vi "ImgCtrl.vi"(7 "Action":enum16{"Initial", "read", "release"}(ring)=enum."release", 10 "GrayImg":T1, 11 "ColorImg":T2) -> (2 "GrayImg":string, 3 "ColorImg":string)   [LabVIEW 2014]
uses:
  Ctrl/ColorImg.ctl
  Ctrl/GrayImg.ctl
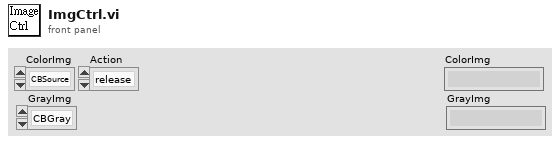
[diagram p1: front panel]
types:
  T1 = typedef "GrayImg.ctl" = enum16{"CBGray"}
  T2 = typedef "ColorImg.ctl" = enum16{"CBSource", "CBShow", "CBToProcess"}
  T3 = typedef "Image Type" = u32
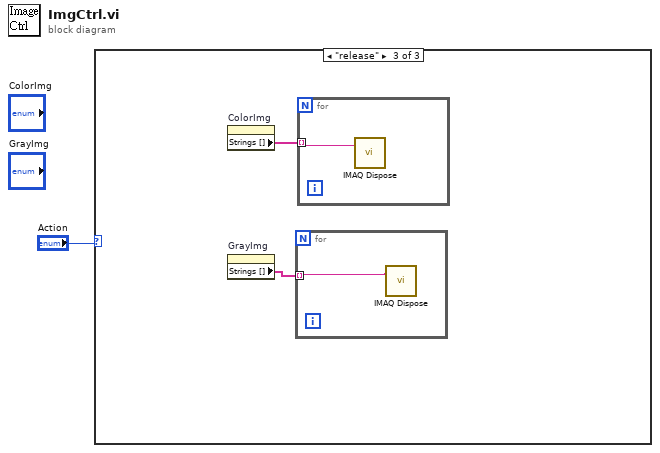
[diagram p0: block diagram]
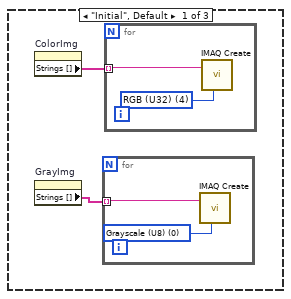
[diagram p2: hidden frame]
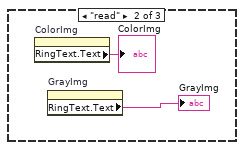
[diagram p3: hidden frame]
diagram:
  n1 = case shown="\"release\"" "Action" {
    frame "Initial", Default {
      n2 = property on="ColorImg" class="Enum (strict)"() -> ("Strings []"=w3:string[])  [unwired: 2 in, 2 out]
      n3 = property on="GrayImg" class="Enum (strict)"() -> ("Strings []"=w2:string[])  [unwired: 2 in, 2 out]
      n4 = for {
        tunnel: w2 -> [w5] mode=indexing
        w4 = T3 0 items=["Grayscale (U8)", "Grayscale (I16)", "Grayscale (SGL)", "Complex (CSG)", "RGB (U32)", "HSL (U32)", "RGB (U64)", "Grayscale (U16)"] ("Image Type")
        n5 = call "IMAQ Create"("Image Name"=w5, "Image Type"=w4) -> ()  [unwired: 3 in, 2 out]
      }
      n6 = for {
        tunnel: w3 -> [w7] mode=indexing
        w6 = T3 4 items=["Grayscale (U8)", "Grayscale (I16)", "Grayscale (SGL)", "Complex (CSG)", "RGB (U32)", "HSL (U32)", "RGB (U64)", "Grayscale (U16)"] ("Image Type")
        n7 = call "IMAQ Create"("Image Name"=w7, "Image Type"=w6) -> ()  [unwired: 3 in, 2 out]
      }
    }
    frame "read" {
      n8 = property on="ColorImg" class="Enum (strict)"() -> ("RingText.Text"=→"ColorImg":string)  [unwired: 2 in, 2 out]
      n9 = property on="GrayImg" class="Enum (strict)"() -> ("RingText.Text"=→"GrayImg":string)  [unwired: 2 in, 2 out]
    }
    frame "release" {
      n10 = property on="ColorImg" class="Enum (strict)"() -> ("Strings []"=w11:string[])  [unwired: 2 in, 2 out]
      n11 = property on="GrayImg" class="Enum (strict)"() -> ("Strings []"=w10:string[])  [unwired: 2 in, 2 out]
      n12 = for {
        tunnel: w10 -> [w12] mode=indexing
        n13 = call "IMAQ Dispose"("Image"=w12) -> ()  [unwired: 5 in, 1 out]
      }
      n14 = for {
        tunnel: w11 -> [w13] mode=indexing
        n15 = call "IMAQ Dispose"("Image"=w13) -> ()  [unwired: 5 in, 1 out]
      }
    }
  }
